vi "NI VeriStand - Open Multiple Waveforms Read Session (DBL).vi"(7 "Communication Properties":T1, 8 "error in (no error)":errorcluster, 11 "DBL Waveform Data References":T2[](array[typedef])) -> (0 "error out":errorcluster, 3 "Multiple Waveforms Read Session (DBL)":refnum<class "Multiple Waveforms Read (DBL).lvclass">)   [LabVIEW 2020, in "NI_VS Custom Device Waveform API.lvlib" / "Multiple Waveforms Read (DBL).lvclass"]
doc: "Opens a session for reading data from or writing data to a specific waveform or waveforms associated with a custom device. You must manually select the instance to use according to the number of waveforms with which you want to interact, whether the data type of the waveforms is DBL or CDB, and whether you want to read or write waveform data."
uses:
  Multiple Waveforms Read (DBL).lvclass
  D:/p4/penguin/lvaddon/Veristand/master/src/LabVIEW/vilib/NI VeriStand/Custom Device Waveform API/Waveform Session.lvclass
  Custom Device API/Waveform Data Reference.ctl
  Communication Properties.ctl
  Access mode.ctl
  Internal Comm Classes/WPL Comm/WPL Comm (1D DBL)/WPL Comm (1D DBL).lvclass
  Multiple Waveforms Read (DBL).lvclass/Multiple Waveforms Read (DBL).ctl
  Waveform Session.lvclass/Waveform Session.ctl
  Waveform Session.lvclass
  NI_VS Custom Device Waveform API.lvlib
  Custom Device API/Custom Device API.lvlib
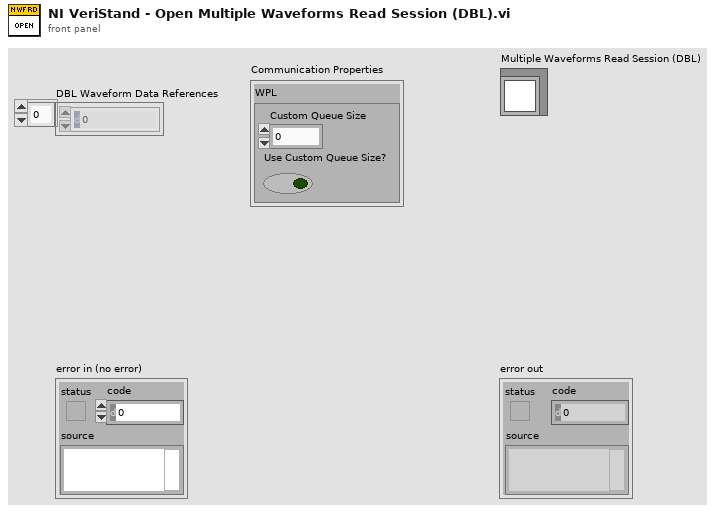
[diagram p1: front panel]
types:
  T1 = typedef "NI_VS Custom Device Waveform API.lvlib/Communication Properties.ctl" = cluster{"WPL":cluster{"Custom Queue Size":i32, "Use Custom Queue Size?":bool}}
  T2 = typedef "Custom Device API.lvlib/Waveform Data Reference.ctl" = i32
  T3 = typedef "NI_VS Custom Device Waveform API.lvlib/Access mode.ctl" = enum16{"Read", "Write"}
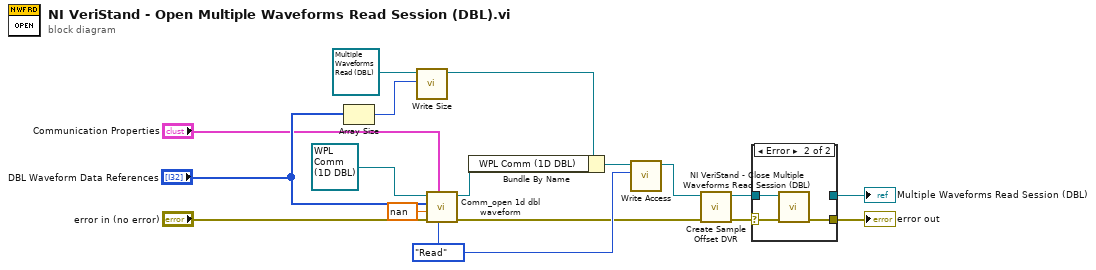
[diagram p0: block diagram]
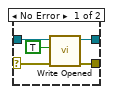
[diagram p2: hidden frame]
diagram:
  w15 = Access_mode."Read" ("Access")
  n1 = Array Size(array="DBL Waveform Data References") -> (size(s)=w8:i32)
  n2 = call "Write Size.vi"("Size"=w8, "Waveform Session in"=refnum<class "Multiple Waveforms Read (DBL).lvclass"> refnum) -> ("Waveform Session out"=w5:refnum<class "Multiple Waveforms Read (DBL).lvclass">)  [unwired: 9 in]
  n3 = call "Comm_open 1d dbl waveform.vi"("Access"=w15, "Communication Properties"="Communication Properties", "error in (no error)"="error in (no error)", "dt"=nan, "WFM Data Ref"="DBL Waveform Data References", "WPL Comm (1D DBL) in"=refnum<class "WPL Comm (1D DBL).lvclass"> refnum ("Internal Comm Classes.lvlib:WPL Comm (1D DBL).lvclass")) -> ("error out"=w13:errorcluster, "WPL Comm (1D DBL) out"=w4:refnum<class "WPL Comm (1D DBL).lvclass">)  [unwired: 4 in]
  n4 = Bundle By Name(cluster=w5, "WPL Comm (1D DBL)"=w4) -> (w3:refnum<class "Multiple Waveforms Read (DBL).lvclass">)
  n5 = call "Write Access.vi"("Access"=w15, "Waveform Session in"=w3) -> ("Waveform Session out"=w10:refnum<class "Multiple Waveforms Read (DBL).lvclass">)  [unwired: 9 in]
  n6 = call "Create Sample Offset DVR.vi"("error in (no error)"=w13, "Waveform Session in"=w10) -> ("error out"=w11:errorcluster, "Waveform Session out"=w12:refnum<class "Multiple Waveforms Read (DBL).lvclass">)  [unwired: 8 in]
  n7 = case shown="Error" w11 {
    selector: w11 -> [w21 w24]
    tunnel: [w21 w23] -> w17
    tunnel: w12 -> [w20 w22]
    tunnel: [w19 _] -> w16
    frame No Error {
      n8 = call "Write Opened.vi"("Opened"=TRUE, "Waveform Session in"=w20) -> ("Waveform Session out"=w19:refnum<class "Multiple Waveforms Read (DBL).lvclass">)  [unwired: 9 in]
    }
    frame Error {
      n9 = call "NI VeriStand - Close Multiple Waveforms Read Session (DBL).vi"("error in (no error)"=w24, "Multiple Waveforms Read Session (DBL)"=w22) -> ("error out"=w23:errorcluster)  [unwired: 9 in]
    }
  }
  "error out" <- w17
  "Multiple Waveforms Read Session (DBL)" <- w16
